vi "Test Helper Loop Cannot Stop Outside Process.vi"(8 "error in (no error)":errorcluster, 11 "Helper Loop Test In":refnum<class "Helper Loop Test.lvclass">) -> (0 "error out":errorcluster, 3 "Helper Loop Test Out":refnum<class "Helper Loop Test.lvclass">)   [LabVIEW 2020, in "Helper Loop Test.lvclass"]
uses:
  Helper Loop Test.lvclass
  Mock Process/Mock Process.lvclass
  C:/Users/anton/Documents/GitHub/Triarc-Framework/source/Framework/Process/Process.lvclass
  C:/Users/anton/Documents/GitHub/Triarc-Framework/source/Framework/Base/Base.lvclass
  C:/Users/anton/Documents/GitHub/Triarc-Framework/source/Framework/Error Handler Interface/Error Handler Interface.lvclass
  C:/Users/anton/Documents/GitHub/Triarc-Framework/source/Framework/Logging/Logging.lvclass
  C:/Users/anton/Documents/GitHub/Triarc-Framework/source/Framework Test/Mock Process/Mock Process.lvclass
  C:/Users/anton/Documents/GitHub/Triarc-Framework/source/Framework/Helper Loop/Helper Loop.lvclass
  Framework/Process/Process.lvclass
  <vilib>/Asteme/LUnit/Test Case.lvclass
  C:/Program Files (x86)/National Instruments/LabVIEW 2020/vi.lib/Asteme/LUnit/Test Case.lvclass
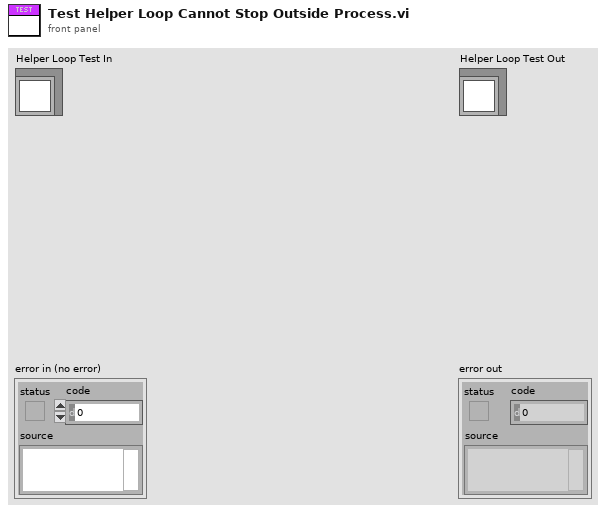
[diagram p1: front panel]
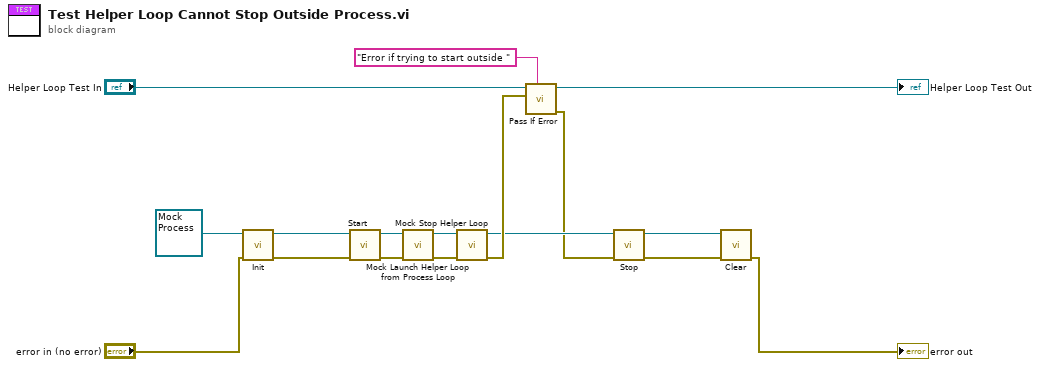
[diagram p0: block diagram]
diagram:
  n1 = call-dynamic "Init.vi"("error in (no error)"="error in (no error)", "Mock Process In"=refnum<class "Mock Process.lvclass"> refnum ("Mock Process.lvclass")) -> ("error out"=w11:errorcluster, "Mock Process Out"=w15:refnum<class "Mock Process.lvclass">)  [unwired: 8 in]
  n2 = call "Start.vi"("error in (no error)"=w11, "Process In"=w15) -> ("error out"=w10:errorcluster, "Process Out"=w2:refnum<class "Mock Process.lvclass">)  [unwired: 8 in]
  n3 = call "Mock Launch Helper Loop from Process Loop.vi"("error in (no error)"=w10, "Mock Process in"=w2) -> ("error out"=w3:errorcluster, "Mock Process out"=w1:refnum<class "Mock Process.lvclass">)  [unwired: 8 in]
  n4 = call "Mock Stop Helper Loop.vi"("error in (no error)"=w3, "Mock Process in"=w1) -> ("error out"=w13:errorcluster, "Mock Process out"=w12:refnum<class "Mock Process.lvclass">)  [unwired: 8 in]
  n5 = call <vilib>:"Pass If Error.vi"("Description"="Error if trying to start outside ", "Assert error"=w13, "Test Case In"="Helper Loop Test In") -> ("error out"=w7:errorcluster, "Test Case Out"=→"Helper Loop Test Out":refnum<class "Helper Loop Test.lvclass">)  [unwired: 7 in]
  n6 = call "Stop.vi"("error in (no error)"=w7, "Process In"=w12) -> ("error out"=w8:errorcluster, "Process Out"=w9:refnum<class "Mock Process.lvclass">)  [unwired: 7 in, 1 out]
  n7 = call-dynamic "Clear.vi"("error in (no error)"=w8, "Mock Process In"=w9) -> ("error out"=→"error out":errorcluster)  [unwired: 9 in]
